vi "read_dust_control_settings.vi"(7 "Settings to be loaded":string, 8 "error in (no error)":errorcluster, 10 "Lower Timestamp Range":timestamp, 11 "Upper Timestamp Range":timestamp) -> (0 "error out":errorcluster, 1 "Array":cluster{"String":string, "Value":string}[](array[cluster]), 3 "Dust Source Array":T1[](array[typedef]) {"Needle Voltage" min=0.0 max=10.0 step=0.01 format="%.2g"; "Y Voltage" min=0.0 max=9.0 step=0.01 format="%.2g"; "X Voltage" min=0.0 max=9.0 step=0.01 format="%.2g"; "Einzel Voltage" min=0.0 max=10.0 step=0.01 format="%.2g"; "Desired Amplitude (V)" min=0.0 max=10.0 step=0.01 format="%5.2f"; "Width (ms) : 0.1" min=0.05 max=5.0 step=0.01 format="%6.2f"; "Frequency" min=1.0 max=100.0 step=0.01 format="%.1f"})   [LabVIEW 2012]
uses:
  dust_soruce_control.ctl
  <vilib>/addons/database/Auxilliary.llb/DB Tools Cursor Type.ctl
  <vilib>/addons/database/Connection.llb/Conn Execute.vi
  <vilib>/addons/database/Recordset.llb/Rec Fetch Recordset Data (R).vi
  <vilib>/addons/database/Recordset.llb/Rec Destroy - Connection.vi
  <vilib>/addons/database/_DB Variant To Data/Database Variant To Data.xnode
  <vilib>/addons/database/NI_Database_API.lvlib
panel:
  out "Settings ID 2":dbl(ring) caption="Settings ID" items=["Auto", "Auto", "Auto", "Auto", "Auto", "Auto", "Auto", "Auto", "Auto", "Auto", "Auto", "Auto", "Auto", "Auto", "Auto", "Auto", "Auto", "Auto", "Auto", "Auto", "Auto test", "Auto", "Automatic Update at  10/19/2012 4:35:52 PM", "Automatic Update at  10/19/2012 4:37:24 PM", "Automatic Update at  10/19/2012 4:37:56 PM", "Automatic Update at  10/19/2012 4:39:59 PM", "Automatic Update at  10/19/2012 4:40:46 PM", "Automatic Update at  10/19/2012 4:43:56 PM", "Automatic Update at  10/19/2012 5:03:34 PM", "Awesome settings that work", "Awesome settings that work", "Automatic Update at  10/19/2012 5:32:08 PM", "Automatic Update at  10/19/2012 5:34:15 PM", "Automatic Update at  10/19/2012 5:39:51 PM", "Working settings", "Working settings", "Working settings", "Working settings", "Working settings", "Automatic Update at  10/22/2012 1:18:52 PM", "Automatic Update at  10/22/2012 1:22:32 PM", "", "Test", "Test", "Automatic Update at  10/22/2012 1:29:56 PM", "Test", "Test 1", "Test 1", "Anna's Settings", "Automatic Update at  10/22/2012 3:57:19 PM", "test of width", "Automatic Update at  10/22/2012 4:02:00 PM", "Automatic Update at  10/22/2012 4:10:30 PM", "Automatic Update at  10/22/2012 4:15:00 PM", "Automatic Update at  10/22/2012 4:38:33 PM", "Automatic Update at  10/22/2012 4:44:48 PM", "Automatic Update at  10/22/2012 4:46:11 PM", "Automatic Update at  10/22/2012 4:51:36 PM", "Automatic Update at  10/22/2012 4:54:36 PM", "Automatic Update at  10/22/2012 4:59:09 PM", "Automatic Update at  10/22/2012 5:01:02 PM", "Automatic Update at  10/22/2012 5:06:29 PM", "Automatic Update at  10/22/2012 5:13:46 PM", "Automatic Update at  10/22/2012 5:18:54 PM", "Automatic Update at  10/22/2012 5:27:58 PM", "Automatic Update at  10/22/2012 5:37:45 PM", "Automatic Update at  10/22/2012 5:39:44 PM", "Automatic Update at  10/22/2012 5:41:21 PM", "Automatic Update at  10/22/2012 5:41:55 PM", "Automatic Update at  10/22/2012 5:43:41 PM", "Automatic Update at  10/22/2012 5:45:31 PM", "Anna's Settings (Updated with working Giraffes)", "Anna's Settings (Updated with working Giraffes)", "Automatic Update at  10/23/2012 1:01:38 PM", "test", "test", "test 1", "test 1", "Automatic Update at  10/23/2012 1:44:56 PM", "Automatic Update at  10/23/2012 1:52:29 PM", "Automatic Update at  10/23/2012 1:59:24 PM", "test 3", "test 4", "Automatic Update at  10/23/2012 2:20:20 PM", "Automatic Update at  10/23/2012 5:53:49 PM", "Anna's Settings", "Anna's Settings1", "test mctesty", "test mctesty", "Automatic Update at  10/24/2012 3:47:44 PM", "Test\"", "Test\"", "this is a \"test\" setting", "Automatic Update at  10/24/2012 4:13:56 PM"]
  out "SQL Query Sintax":string
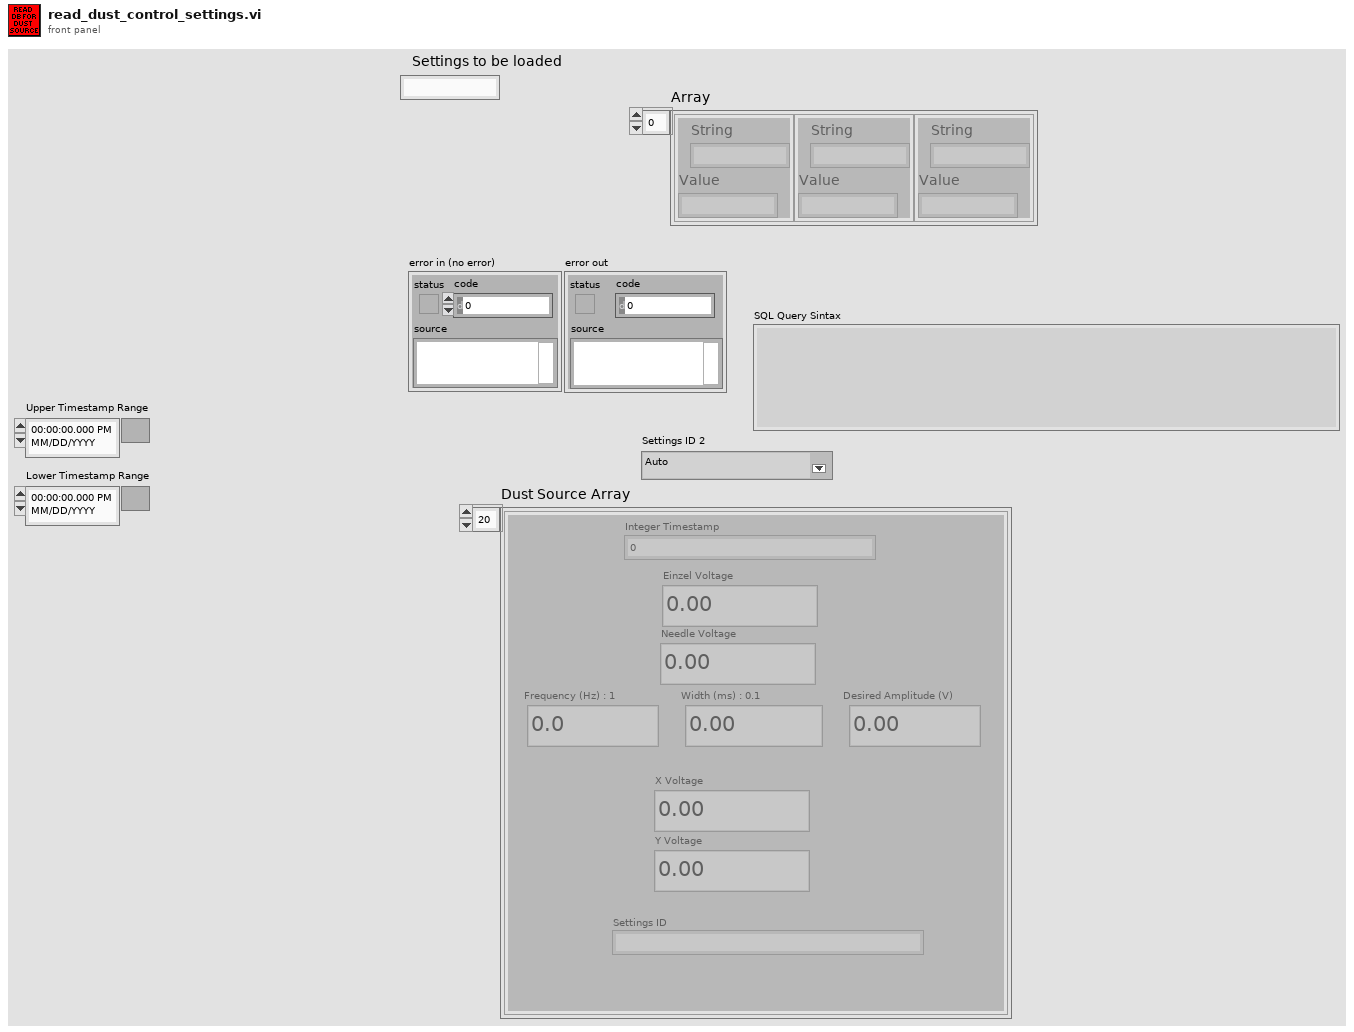
[diagram p1: front panel]
types:
  T1 = typedef "dust_soruce_control.ctl" = cluster{"Integer Timestamp":u64, "Einzel Voltage":dbl, "Needle Voltage":dbl, "Frequency":dbl, "Width (ms) : 0.1 ":dbl, "Desired Amplitude (V)":dbl, "X Voltage":dbl, "Y Voltage":dbl, "Settings ID":string, "ID#":dbl}
  T2 = typedef "NI_Database_API.lvlib/DB Tools Cursor Type.ctl" = enum16{"forward-only", "keyset", "dynamic", "static"}
  T3 = typedef "NI_Database_API.lvlib/Conn ObjectReference.ctl" = refnum<k1>
  T4 = typedef "NI_Database_API.lvlib/Rec ObjectReference.ctl" = refnum<k1>
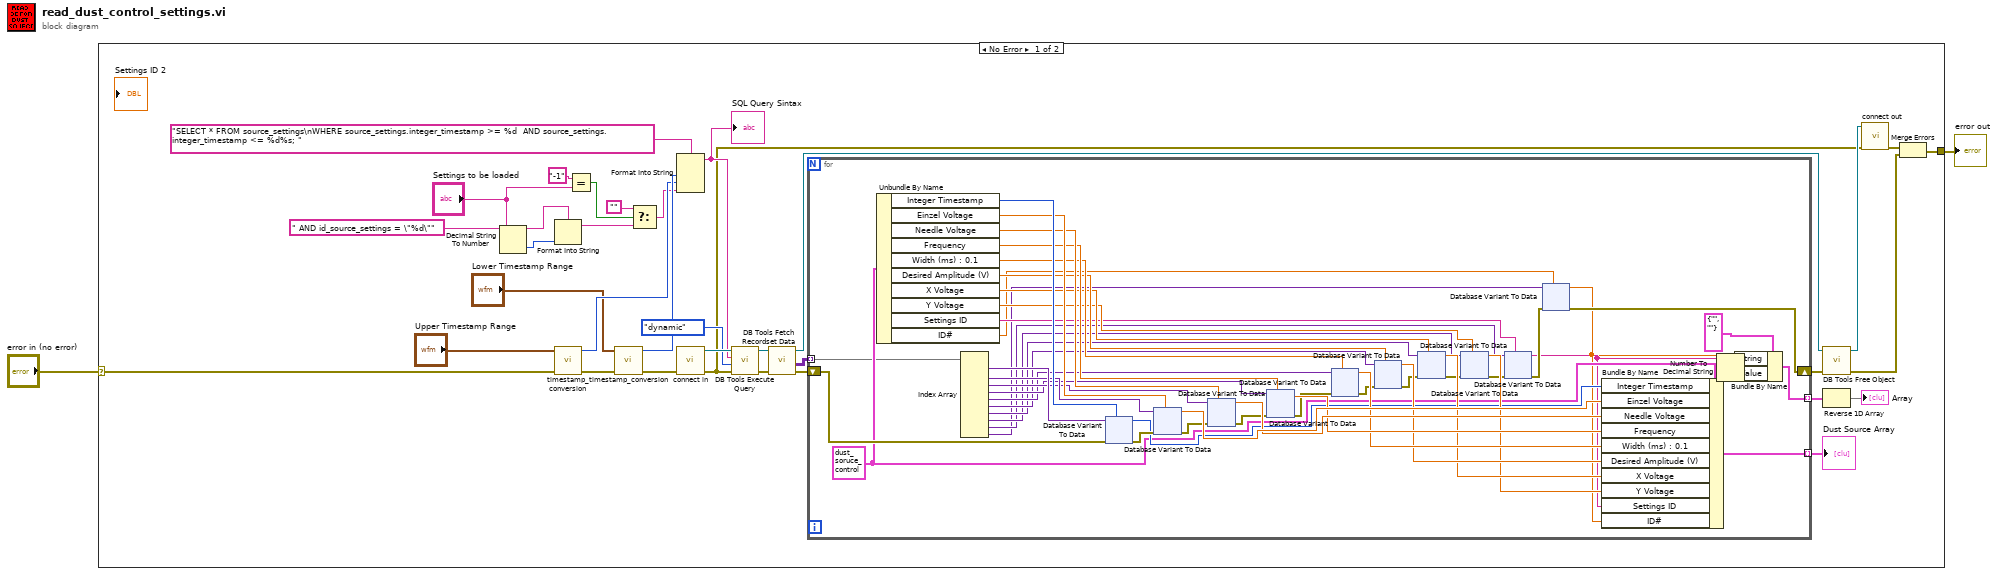
[diagram p0: block diagram]
diagram:
  n1 = case shown="No Error" "error in (no error)" {
    selector: "error in (no error)" -> [w26 w403]
    tunnel: [w6 w403] -> w1
    frame No Error {
      n2 = Decimal String To Number(string="Settings to be loaded") -> (number=w3:i32)  [unwired: 2 in, 1 out]
      n3 = Format Into String(format string=" AND id_source_settings = \"%d\"" ("string"), w3) -> (resulting string=w22:string)  [unwired: 2 in, 1 out]
      n4 = call "timestamp_conversion.vi"("error in (no error)"=w26, "Time Stamp"="Upper Timestamp Range") -> ("error out"=w27:errorcluster, "Integer Time"=w19:i64)  [unwired: 7 in]
      n5 = Equal?(x="-1" ("Settings to be loaded"), y="Settings to be loaded") -> (x = y?=w28:bool)
      n6 = call "timestamp_conversion.vi"("error in (no error)"=w27, "Time Stamp"="Lower Timestamp Range") -> ("error out"=w24:errorcluster, "Integer Time"=w20:i64)  [unwired: 7 in]
      n7 = Select(t="", s=w28, f=w22) -> (s? t:f=w12:string)
      n8 = Format Into String(format string="SELECT * FROM source_settings\nWHERE source_settings.integer_timestamp >= %d  AND source_settings.integer_timestamp <= %d%s; " ("string"), w20, w19, w12) -> (resulting string=w17:string)  [unwired: 2 in, 1 out]
      "SQL Query Sintax" <- w17
      n9 = call "connect in.vi"("error in (no error)"=w24) -> ("error out"=w4:errorcluster, "Database Connection"=w30:T3)  [unwired: 6 in, 1 out]
      n10 = call-poly <vilib>:"DB Tools Execute Query.vi"("error in (no error)"=w4, "cursor type"=DB_Tools_Cursor_Type."dynamic", "SQL query"=w17, "connection reference"=w30) -> ("error out"=w34:errorcluster, "recordset reference"=w35:T4)  [unwired: 4 in]
      n11 = call-poly <vilib>:"DB Tools Fetch Recordset Data.vi"("error in (no error)"=w34, "recordset reference"=w35) -> ("error out"=w32:errorcluster, "recordset data"=w25:variant[][], "recordset reference out"=w33:T4)  [unwired: 3 in]
      n12 = for {
        tunnel: w25 -> [w63] mode=indexing
        shift-right: [w43] -> w31
        shift-left: w32 -> [w82]
        tunnel: [w66] -> w10 mode=indexing
        tunnel: [w39] -> w9 mode=indexing
        w64 = T1 {"Integer Timestamp"=0, "Einzel Voltage"=0.0, "Needle Voltage"=0.0, "Frequency"=1.0, "Width (ms) : 0.1 "=0.05, "Desired Amplitude (V)"=0.0, "X Voltage"=0.0, "Y Voltage"=0.0, "Settings ID"="", "ID#"=0.0} ("Dust Source Controls")
        n13 = Unbundle By Name(w64) -> ("Integer Timestamp"=w62:u64, "Einzel Voltage"=w60:dbl, "Needle Voltage"=w58:dbl, "Frequency"=w56:dbl, "Width (ms) : 0.1"=w54:dbl, "Desired Amplitude (V)"=w51:dbl, "X Voltage"=w49:dbl, "Y Voltage"=w48:dbl, "Settings ID"=w46:string, "ID#"=w41:dbl)
        n14 = Index Array(array=w63) -> (element #1=w61:variant, element #2=w59:variant, element #3=w57:variant, element #4=w55:variant, element #5=w53:variant, element #6=w52:variant, element #7=w50:variant, element #8=w47:variant, element #9=w45:variant, element #10=w42:variant)  [unwired: 10 in]
        n15 = xnode "Database Variant To Data"("database variant"=w61, "error in"=w82, "type"=w62) -> ("data"=w65:u64, "error out"=w80:errorcluster)
        n16 = xnode "Database Variant To Data"("database variant"=w59, "error in"=w80, "type"=w60) -> ("data"=w81:dbl, "error out"=w78:errorcluster)
        n17 = xnode "Database Variant To Data"("database variant"=w57, "error in"=w78, "type"=w58) -> ("data"=w79:dbl, "error out"=w76:errorcluster)
        n18 = xnode "Database Variant To Data"("database variant"=w55, "error in"=w76, "type"=w56) -> ("data"=w77:dbl, "error out"=w74:errorcluster)
        n19 = xnode "Database Variant To Data"("database variant"=w53, "error in"=w74, "type"=w54) -> ("data"=w75:dbl, "error out"=w73:errorcluster)
        n20 = xnode "Database Variant To Data"("database variant"=w52, "error in"=w73, "type"=w51) -> ("data"=w72:dbl, "error out"=w70:errorcluster)
        n21 = xnode "Database Variant To Data"("database variant"=w50, "error in"=w70, "type"=w49) -> ("data"=w71:dbl, "error out"=w68:errorcluster)
        n22 = xnode "Database Variant To Data"("database variant"=w47, "error in"=w68, "type"=w48) -> ("data"=w69:dbl, "error out"=w67:errorcluster)
        n23 = xnode "Database Variant To Data"("database variant"=w45, "error in"=w67, "type"=w46) -> ("data"=w38:string, "error out"=w44:errorcluster)
        n24 = xnode "Database Variant To Data"("database variant"=w42, "error in"=w44, "type"=w41) -> ("data"=w37:dbl, "error out"=w43:errorcluster)
        n25 = Bundle By Name(cluster=w64, "Integer Timestamp"=w65, "Einzel Voltage"=w81, "Needle Voltage"=w79, "Frequency"=w77, "Width (ms) : 0.1"=w75, "Desired Amplitude (V)"=w72, "X Voltage"=w71, "Y Voltage"=w69, "Settings ID"=w38, "ID#"=w37) -> (w66:T1)
        n26 = Number To Decimal String(number=w37) -> (decimal integer string=w36:string)  [unwired: 1 in]
        n27 = Bundle By Name(cluster=cluster{"String":string, "Value":string} {"String"="", "Value"=""}, "String"=w38, "Value"=w36) -> (w39:cluster{"String":string, "Value":string})
      }
      "Dust Source Array" <- w10
      n28 = call-poly <vilib>:"DB Tools Free Object.vi"("error in (no error)"=w31, "recordset reference"=w33) -> ("error out"=w5:errorcluster, "connection reference"=w29:T3)  [unwired: 8 in]
      n29 = Reverse 1D Array(array=w9) -> (reversed array=→"Array":cluster{"String":string, "Value":string}[])
      n30 = call "connect out.vi"("error in (no error)"=w4, "connection reference"=w29) -> ("error out"=w7:errorcluster)  [unwired: 9 in]
      n31 = Merge Errors(w7, w5) -> (w6:errorcluster)
    }
    frame Error {
    }
  }
  "error out" <- w1
